vi "Get GObj UID.vi"(8 "错误输入（无错误）":errorcluster, 11 "GObj Ref  In":refnum<vi>) -> (0 "错误输出":errorcluster, 2 "UID":i32, 3 "GObj Ref Out":refnum<vi>)   [LabVIEW 2012, in "CtrlRef.lvlib"]
uses:
  CtrlRef.lvlib
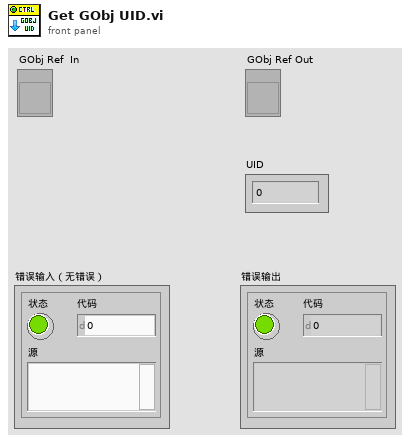
[diagram p1: front panel]
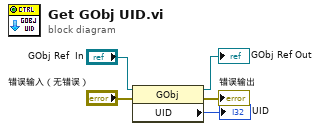
[diagram p0: block diagram]
diagram:
  n1 = property class="GObj"(reference="GObj Ref  In", error in="错误输入（无错误）") -> (reference out=→"GObj Ref Out":refnum<vi>, error out=→"错误输出":errorcluster, "UID"=→"UID":i32)
